vi "Check login.vi"(7 "Data I/p":string[][](array[string]), 8 "User Type":string, 9 "Password":string, 10 "User Name":string) -> (1 "Login Type":string, 2 "User Name 2":string, 3 "OK":bool)   [LabVIEW 2024]
uses:
  Instance           1 19Saved   Check login .vi
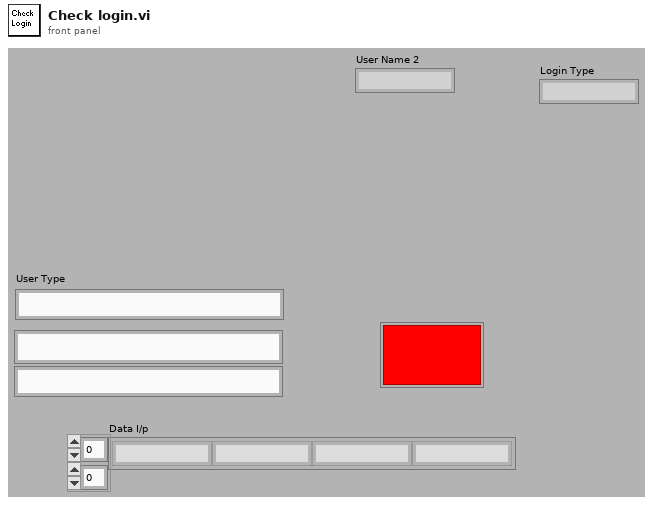
[diagram p1: front panel]
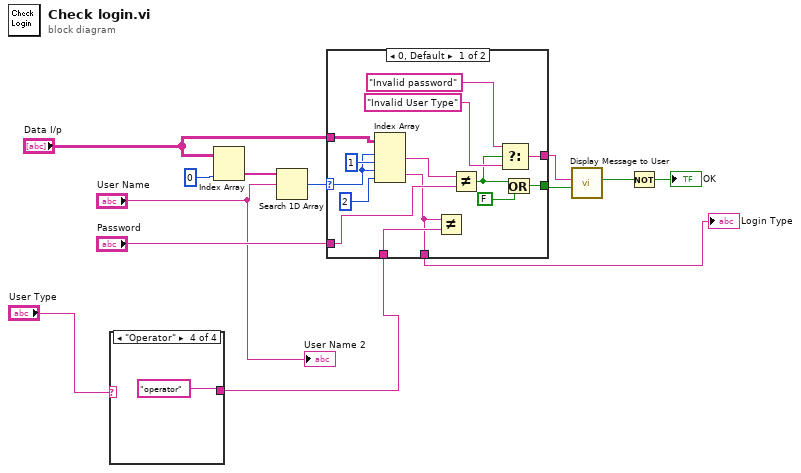
[diagram p0: block diagram]
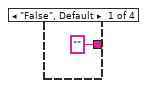
[diagram p2: hidden frame]
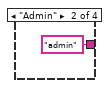
[diagram p3: hidden frame]
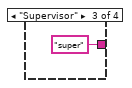
[diagram p4: hidden frame]
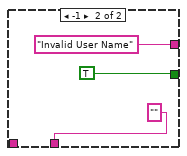
[diagram p5: hidden frame]
diagram:
  n1 = case shown="\"Operator\"" "User Type" {
    tunnel: ["" ("Message") "admin" ("Message") "super" ("Message") "operator" ("Message")] -> w2
    frame "False", Default {
    }
    frame "Admin" {
    }
    frame "Supervisor" {
    }
    frame "Operator" {
    }
  }
  n2 = Index Array(array="Data I/p", index (col)=0 ("index (row)")) -> (element=w9:string[])  [unwired: 1 in]
  n3 = Search 1D Array(1D array=w9, element="User Name") -> (index of element=w7:i32)  [unwired: 1 out]
  n4 = case shown="0, Default" w7 {
    selector: w7 -> [w27 _]
    tunnel: "Data I/p" -> [w31 _]
    tunnel: "Password" -> [w28 _]
    tunnel: [w24 TRUE] -> w6
    tunnel: [w21 "Invalid User Name" ("Message")] -> w5
    tunnel: w2 -> [w25 _]
    tunnel: [w18 "" ("username")] -> w1
    frame 0, Default {
      n5 = Index Array(array=w31, index (row) #1=w27, index (col) #1=1 ("disabled index (col)"), index (row) #2=w27, index (col) #2=2 ("disabled index (col)")) -> (element #1=w29:string, element #2=w18:string)
      n6 = Not Equal?(x=w18, y=w25) -> ()  [unwired: 1 out]
      n7 = Not Equal?(x=w29, y=w28) -> (x != y?=w20:bool)
      n8 = Select(t="Invalid password" ("Message"), s=w20, f="Invalid User Type" ("Message")) -> (s? t:f=w21:string)
      n9 = Or(x=w20, y=FALSE) -> (x .or. y?=w24:bool)
    }
    frame -1 {
    }
  }
  "Login Type" <- w1
  n10 = call "Display Message to User"("Enable"=w6, "Message"=w5) -> ("OK"=w4:bool)  [unwired: 1 in, 8 out]
  n11 = Not(x=w4) -> (.not. x?=→"OK":bool)
  "User Name 2" <- "User Name"
